vi "传感器数据.vi"() -> (0 "电机角度":sgl format="%#.3f", 1 "拉压力":sgl format="%#.3f", 2 "扭矩":sgl format="%#.3f", 3 "电缸位移":sgl format="%#.3f", 4 "电缸自带压力":sgl format="%#.3f")   [LabVIEW 2020]
uses:
  Libraries/S7/S7.lvlib
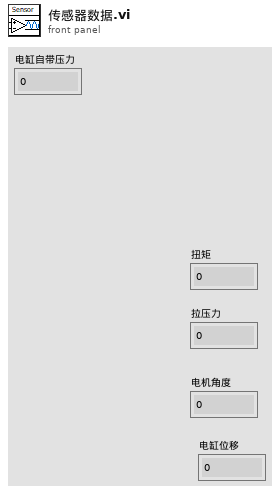
[diagram p1: front panel]
types:
  T1 = typedef "S7.lvlib/Read_Data (Reply Payload)--cluster.ctl" = cluster{"读取成功":bool, "数据":u32[], "Read_Data_error":errorcluster}
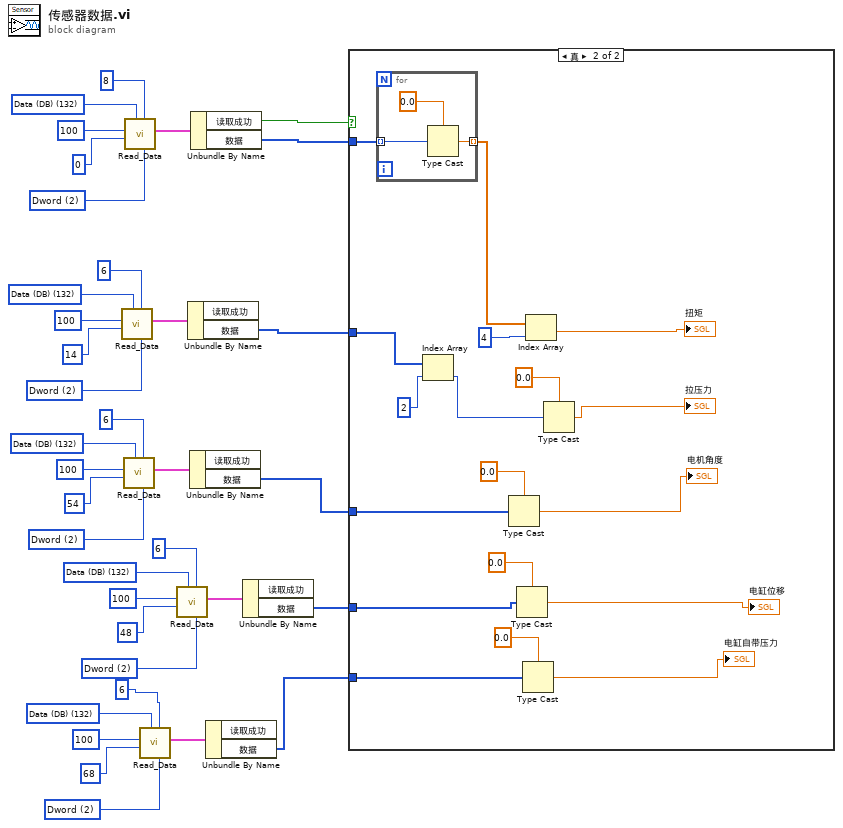
[diagram p0: block diagram]
diagram:
  w7 = u16 2 items=["byte", "word", "Dword"] ("数据类型")
  w5 = u8 132 items=["I/O (P)"=128, "Input (I)"=129, "Output (Q)"=130, "Bit Memory (M)"=131, "Data (DB)"=132, "Instance Data (DI)"=133, "Local Data (L)"=134, "Predecessor Local Data (VL)"=135] ("寄存器类型")
  w9 = u16 2 items=["byte", "word", "Dword"] ("数据类型")
  w12 = u8 132 items=["I/O (P)"=128, "Input (I)"=129, "Output (Q)"=130, "Bit Memory (M)"=131, "Data (DB)"=132, "Instance Data (DI)"=133, "Local Data (L)"=134, "Predecessor Local Data (VL)"=135] ("寄存器类型")
  w18 = u16 2 items=["byte", "word", "Dword"] ("数据类型")
  w19 = u8 132 items=["I/O (P)"=128, "Input (I)"=129, "Output (Q)"=130, "Bit Memory (M)"=131, "Data (DB)"=132, "Instance Data (DI)"=133, "Local Data (L)"=134, "Predecessor Local Data (VL)"=135] ("寄存器类型")
  w26 = u16 2 items=["byte", "word", "Dword"] ("数据类型")
  w25 = u8 132 items=["I/O (P)"=128, "Input (I)"=129, "Output (Q)"=130, "Bit Memory (M)"=131, "Data (DB)"=132, "Instance Data (DI)"=133, "Local Data (L)"=134, "Predecessor Local Data (VL)"=135] ("寄存器类型")
  w33 = u16 2 items=["byte", "word", "Dword"] ("数据类型")
  w34 = u8 132 items=["I/O (P)"=128, "Input (I)"=129, "Output (Q)"=130, "Bit Memory (M)"=131, "Data (DB)"=132, "Instance Data (DI)"=133, "Local Data (L)"=134, "Predecessor Local Data (VL)"=135] ("寄存器类型")
  n1 = call "Read_Data.vi"("数据类型"=w26, "读取长度"=u16 6, "寄存器类型"=w25, "起始地址"=u32 14, "DB #"=u16 100) -> ("Reply Payload"=w28:T1)  [unwired: 4 in, 2 out]
  n2 = call "Read_Data.vi"("数据类型"=w18, "读取长度"=u16 6, "寄存器类型"=w19, "起始地址"=u32 54, "DB #"=u16 100) -> ("Reply Payload"=w16:T1)  [unwired: 4 in, 2 out]
  n3 = call "Read_Data.vi"("数据类型"=w33, "读取长度"=u16 8, "寄存器类型"=w34, "起始地址"=u32 0, "DB #"=u16 100) -> ("Reply Payload"=w31:T1)  [unwired: 4 in, 2 out]
  n4 = call "Read_Data.vi"("数据类型"=w7, "读取长度"=u16 6, "寄存器类型"=w5, "起始地址"=u32 68, "DB #"=u16 100) -> ("Reply Payload"=w3:T1)  [unwired: 4 in, 2 out]
  n5 = call "Read_Data.vi"("数据类型"=w9, "读取长度"=u16 6, "寄存器类型"=w12, "起始地址"=u32 48, "DB #"=u16 100) -> ("Reply Payload"=w14:T1)  [unwired: 4 in, 2 out]
  n6 = Unbundle By Name(w28) -> ("数据"=w22:u32[])  [unwired: 1 out]
  n7 = Unbundle By Name(w16) -> ("数据"=w15:u32[])  [unwired: 1 out]
  n8 = Unbundle By Name(w31) -> ("读取成功"=w29:bool, "数据"=w30:u32[])
  n9 = Unbundle By Name(w3) -> ("数据"=w1:u32[])  [unwired: 1 out]
  n10 = Unbundle By Name(w14) -> ("数据"=w8:u32[])  [unwired: 1 out]
  n11 = case shown="真" w29 {
    tunnel: w30 -> [_ w54]
    tunnel: w22 -> [_ w50]
    tunnel: w15 -> [_ w44]
    tunnel: w8 -> [_ w41]
    tunnel: w1 -> [_ w38]
    frame False {
    }
    frame True {
      n12 = for {
        tunnel: w54 -> [w56] mode=indexing
        tunnel: [w55] -> w53 mode=indexing
        n13 = Type Cast(type=sgl 0.0, x=w56) -> (*(type *) &x=w55:sgl)
      }
      n14 = Index Array(array=w50, index=2 ("索引")) -> (element=w47:u32)
      n15 = Type Cast(type=sgl 0.0, x=w44) -> (*(type *) &x=→"电机角度":sgl)
      n16 = Type Cast(type=sgl 0.0, x=w41) -> (*(type *) &x=→"电缸位移":sgl)
      n17 = Type Cast(type=sgl 0.0, x=w38) -> (*(type *) &x=→"电缸自带压力":sgl)
      n18 = Index Array(array=w53, index=4 ("索引")) -> (element=→"扭矩":sgl)
      n19 = Type Cast(type=sgl 0.0, x=w47) -> (*(type *) &x=→"拉压力":sgl)
    }
  }
